vi "FGV_TENMAread.vi"(8 "errin":errorcluster caption="entrée d'erreur (pas d'erreur)", 10 "Énum":T1, 11 "Numeric input":dbl) -> (0 "errout":errorcluster caption="sortie d'erreur", 3 "Numeric output":dbl)   [LabVIEW 2020]
uses:
  ZEN8 Semi Auto EMC/OP700/SubVI/FGV/FGV_Enum.ctl
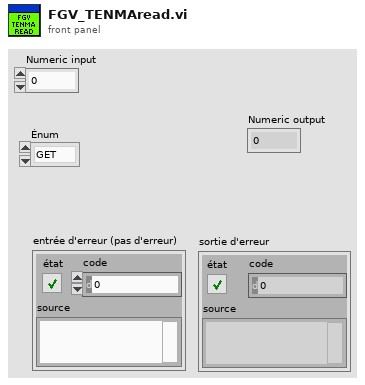
[diagram p1: front panel]
types:
  T1 = typedef "FGV_Enum.ctl" = enum16{"GET", "SET"}
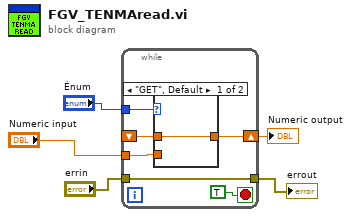
[diagram p0: block diagram]
diagram:
  n1 = while {
    tunnel: "Énum" -> [w10]
    shift-right: [w9] -> w1
    shift-left: _ -> [w8]
    tunnel: "errin" -> [w7]
    tunnel: [w7] -> w3
    tunnel: "Numeric input" -> [w6]
    stop <- TRUE stop-if-true
    n2 = case shown="\"GET\", Default" w10 {
      tunnel: [w12 w13] -> w9
      tunnel: w8 -> [w12 _]
      tunnel: w6 -> [_ w13]
      frame "GET", Default {
      }
      frame "SET" {
      }
    }
  }
  "errout" <- w3
  "Numeric output" <- w1
